vi "Exercise1.12-State Indicator-S1.vi"() -> ()   [LabVIEW 2013]
panel:
  out "output2":dbl
  out "output1":dbl
  in  "input":dbl
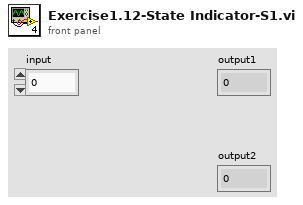
[diagram p1: front panel]
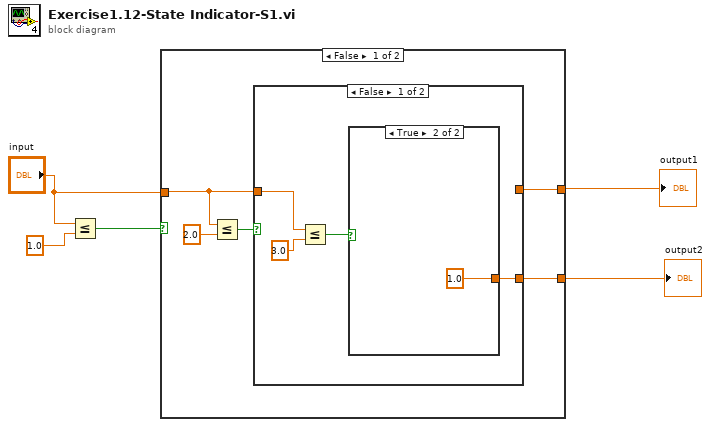
[diagram p0: block diagram]
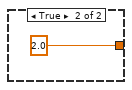
[diagram p3: hidden frame]
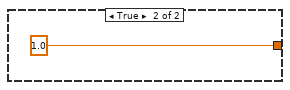
[diagram p4: hidden frame]
diagram:
  n1 = Less Or Equal?(x="input", y=1.0) -> (x <= y?=w4:bool)
  n2 = case shown="False" w4 {
    tunnel: [w7 1.0] -> w3
    tunnel: "input" -> [w8 _]
    tunnel: [w6 _] -> w1
    frame False {
      n3 = Less Or Equal?(x=w8, y=2.0) -> (x <= y?=w9:bool)
      n4 = case shown="False" w9 {
        tunnel: w8 -> [w13 _]
        tunnel: [_ 2.0] -> w7
        tunnel: [w11 _] -> w6
        frame False {
          n5 = Less Or Equal?(x=w13, y=3.0) -> (x <= y?=w14:bool)
          n6 = case shown="True" w14 {
            tunnel: [_ 1.0] -> w11
            frame False {
            }
            frame True {
            }
          }
        }
        frame True {
        }
      }
    }
    frame True {
    }
  }
  "output1" <- w3
  "output2" <- w1
